vi "Check Password.vi"(8 "error in (no error)":errorcluster, 11 "[V] Login in":refnum<class "[V] Login.lvclass">) -> (0 "error out":errorcluster, 2 "password":string, 3 "[V] Login out":refnum<class "[V] Login.lvclass">)   [LabVIEW 2020, in "[V] Login.lvlib" / "[V] Login.lvclass"]
uses:
  [V] Login.lvclass
  [V] Login.lvclass/[V] Login.ctl
  <vilib>/YU/YU-Encrypt/MD5/MD5.lvclass
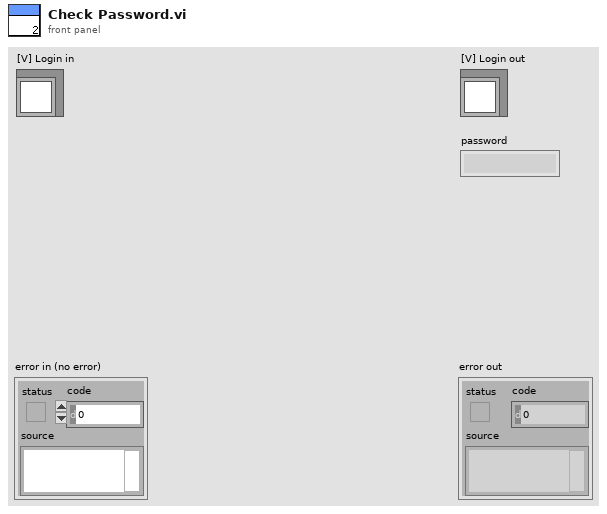
[diagram p1: front panel]
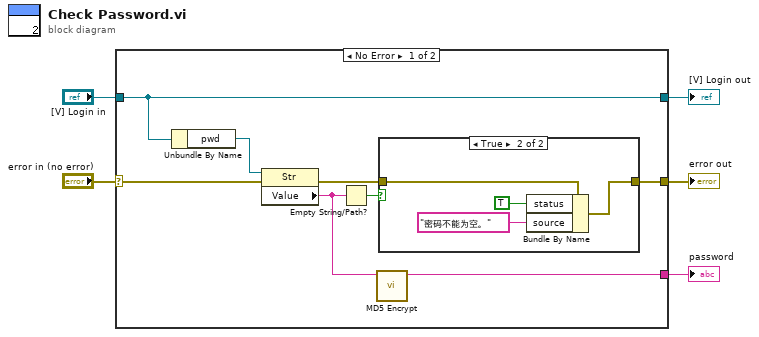
[diagram p0: block diagram]
diagram:
  n1 = case shown="No Error" "error in (no error)" {
    selector: "error in (no error)" -> [w12 w20]
    tunnel: [w8 w20] -> w4
    tunnel: [w13 w19] -> w2
    tunnel: "[V] Login in" -> [w13 w19]
    tunnel: [w6 _] -> w1
    frame No Error {
      n2 = Unbundle By Name(w13) -> ("pwd"=w11:refnum<vi>)
      n3 = property class="Str"(reference=w11, error in=w12) -> (error out=w9:errorcluster, "Value"=w7:string)  [unwired: 1 out]
      n4 = Empty String/Path?(string/path=w7) -> (empty?=w10:bool)
      n5 = call <vilib>:"MD5 Encrypt.vi"("data"=w7) -> ("encrypted data"=w6:string)  [unwired: 9 in, 1 out]
      n6 = case shown="True" w10 {
        tunnel: w9 -> [w14 w18]
        tunnel: [w14 w15] -> w8
        frame False {
        }
        frame True {
          n7 = Bundle By Name(cluster=w18, "status"=TRUE, "source"="密码不能为空。") -> (w15:errorcluster)
        }
      }
    }
    frame Error {
    }
  }
  "error out" <- w4
  "[V] Login out" <- w2
  "password" <- w1
